vi "ATCpilot.vi"() -> ()   [LabVIEW 2014]
doc: "ATC app"
uses:
  <vilib>/Utility/config.llb/NI_LVConfig.lvlib
  <vilib>/Utility/config.llb/Read Key (String).vi
panel:
  in  "정지":bool
  in  "정보1":bool
  in  "도움말":bool
  in  "?":bool
  in  "?":bool
  in  "탭":T1(tab)
  in  "메모":string="필요한 메모를 할수 있습니다. "
  in  "SID&RadarVector. 2":string="SID&RadarVector. "
  in  "인사말":string="인사말"
  in  "CD관제기관":string="관제기관"
  in  "콜사인":string="콜사인\n콜사인\n콜사인"
  in  "도착공항":string="도착공항"
  in  "SID&RadarVector":string="SID&RadarVector"
  in  "비행고도":string="비행고도"
  in  "인사말2":string="인사말"
  in  "콜사인2":string="콜사인"
  in  "콜사인3":string="콜사인"
  in  "콜사인4":string="콜사인"
  in  "콜사인5":string="콜사인"
  in  "콜사인6":string="콜사인"
  in  "도착공항2":string="도착공항"
  in  "제한고도":string="제한고도"
  in  "비행고도2":string="비행고도"
  in  "D접속주파수":string="접속주파수"
  in  "스콱번호":string="스콱번호"
  in  "도착공항3":string="도착공항"
  in  "SID&RadarVector. 3":string="SID&RadarVector. "
  in  "제한고도2":string="제한고도"
  in  "비행고도3":string="비행고도"
  in  "D접속주파수2":string="접속주파수"
  in  "스콱번호2":string="스쾃번호"
  in  "콜사인7":string="콜사인"
  in  "콜사인8":string="콜사인"
  in  "G관제기관":string="관제기관"
  in  "G접속주파수2":string="접속주파수"
  in  "G관제기관2":string="관제기관"
  in  "G접속주파수":string="접속주파수"
  in  "콜사인9":string="콜사인"
  in  "유도로 2":string="유도로"
  in  "유도로":string="유도로"
  in  "방향 2":string="방향"
  in  "방향":string="방향"
  in  "메모2":string="필요한 메모를 할수 있습니다. "
  in  "T관제기관2":string="관제기관"
  in  "콜사인24":string="콜사인"
  in  "T접속주파수2":string="접속주파수"
  in  "T접속주파수":string="접속주파수"
  in  "T관제기관":string="관제기관"
  in  "콜사인23":string="콜사인"
  in  "활주로9":string="활주로"
  in  "G관제기관4":string="관제기관"
  in  "콜사인22":string="콜사인"
  in  "콜사인21":string="콜사인"
  in  "콜사인20":string="콜사인"
  in  "콜사인19":string="콜사인"
  in  "활주로8":string="활주로"
  in  "활주로7":string="활주로"
  in  "콜사인17":string="콜사인"
  in  "활주로6":string="활주로"
  in  "콜사인18":string="콜사인"
  in  "활주로5":string="활주로"
  in  "콜사인16":string="콜사인"
  in  "활주로4":string="활주로"
  in  "콜사인15":string="콜사인"
  in  "활주로3":string="활주로"
  in  "콜사인14":string="콜사인"
  in  "콜사인13":string="콜사인"
  in  "현재기압2":string="현재기압"
  in  "출발공항":string="출발공항"
  in  "활주로2":string="활주로"
  in  "현재기압":string="현재기압"
  in  "출발공항2":string="출발공항"
  in  "활주로1":string="활주로"
  in  "콜사인12":string="콜사인"
  in  "콜사인11":string="콜사인"
  in  "G관제기관3":string="관제기관"
  in  "인사3":string="인사"
  in  "콜사인34 2":string="콜사인"
  in  "D관제기관2":string="관제기관"
  in  "D관제기관":string="관제기관"
  in  "T관제기관3":string="관제기관"
  in  "메모3":string="필요한 메모를 할수 있습니다. "
  in  "인사4":string="인사"
  in  "콜사인25":string="콜사인"
  in  "활주로10":string="활주로"
  in  "콜사인26":string="콜사인"
  in  "바람방향":string="바람방향"
  in  "풍속":string="풍속"
  in  "콜사인28":string="콜사인"
  in  "활주로13":string="활주로"
  in  "콜사인29":string="콜사인"
  in  "활주로12":string="활주로"
  in  "콜사인30":string="콜사인"
  in  "활주로14":string="활주로"
  in  "콜사인31":string="콜사인"
  in  "활주로15":string="활주로"
  in  "T관제기관4":string="관제기관"
  in  "콜사인32":string="콜사인"
  in  "현재고도":string="현재고도"
  in  "허가고도":string="허가고도"
  in  "콜사인33":string="콜사인"
  in  "접속주파수":string="접속주파수"
  in  "콜사인34":string="콜사인"
  in  "접속주파수2":string="접속주파수"
  in  "순항고도or이니셜고도":string="순항고도or이니셜고도"
  in  "D관제기관5":string="관제기관"
  in  "메모 4":string="필요한 메모를 할수 있습니다. "
  in  "인사5":string="인사"
  in  "D관제기관3":string="관제기관"
  in  "콜사인35":string="콜사인"
  in  "현재고도A":string="현재고도"
  in  "콜사인36":string="콜사인"
  in  "D관제기관4":string="관제기관"
  in  "허가고도4":string="허가고도"
  in  "허가고도5":string="허가고도"
  in  "콜사인37":string="콜사인"
  in  "콜사인38":string="콜사인"
  in  "허가고도6":string="허가고도"
  in  "허가고도7":string="허가고도"
  in  "콜사인39":string="콜사인"
  in  "콜사인40":string="콜사인"
  in  "C관제기관":string="관제기관"
  in  "A접속주파수":string="접속주파수"
  in  "C관제기관2":string="관제기관"
  in  "A접속주파수2":string="접속주파수"
  in  "콜사인41":string="콜사인"
  in  "콜사인38 2":string="콜사인"
  in  "D관제기관6":string="관제기관"
  in  "허가고도6 2":string="허가고도"
  in  "허가고도6 3":string="허가고도"
  in  "콜사인39 2":string="콜사인"
  in  "메모5":string="필요한 메모를 할수 있습니다. "
  in  "인사말 2":string="인사말"
  in  "허가고도 2":string="허가고도"
  in  "지점":string="지점"
  in  "허가고도7 2":string="허가고도"
  in  "콜사인38 3":string="콜사인"
  in  "콜사인39 3":string="콜사인"
  in  "허가고도7 3":string="허가고도"
  in  "지점 2":string="지점"
  in  "메모6":string="필요한 메모를 할수 있습니다. "
  in  "A관제기관3":string="관제기관"
  in  "콜사인46":string="콜사인"
  in  "날시정보":string="날시정보"
  in  "고도":string="고도"
  in  "콜사인47":string="콜사인"
  in  "A관제기관4":string="관제기관"
  in  "L활주로":string="활주로"
  in  "도착공항4":string="도착공항"
  in  "현재기압":string="현재기압"
  in  "콜사인48":string="콜사인"
  in  "A관제기관5":string="관제기관"
  in  "L활주로":string="활주로"
  in  "도착공항5":string="도착공항"
  in  "현재기압":string="현재기압"
  in  "콜사인49":string="콜사인"
  in  "고도":string="고도"
  in  "콜사인50":string="콜사인"
  in  "고도":string="고도"
  in  "콜사인51":string="콜사인"
  in  "고도":string="고도"
  in  "고도":string="고도"
  in  "콜사인52":string="콜사인"
  in  "콜사인53":string="콜사인"
  in  "A관제기관":string="관제기관"
  in  "풍속":string="풍속"
  in  "바람방향":string="바람방향"
  in  "L활주로3":string="활주로"
  in  "콜사인54":string="콜사인"
  in  "L활주로":string="활주로"
  in  "콜사인55":string="콜사인"
  in  "A관제기관2":string="관제기관"
  in  "L활주로":string="활주로"
  in  "ILS":string="주파수(ils)"
  in  "콜사인56":string="콜사인"
  in  "L활주로6":string="활주로"
  in  "ILS2":string="주파수(ils)"
  in  "콜사인57":string="콜사인"
  in  "T관제기관":string="관제기관"
  in  "T접속주파수":string="접속주파수"
  in  "콜사인58":string="콜사인"
  in  "콜사인59":string="콜사인"
  in  "관제기관":string="관제기관"
  in  "T접속주파수":string="접속주파수"
  in  "메모7":string="필요한 메모를 할수 있습니다. "
  in  "바람방향":string="바람방향"
  in  "관제기관":string="관제기관"
  in  "콜사인60":string="콜사인"
  in  "L활주로7":string="활주로"
  in  "콜사인61":string="콜사인"
  in  "풍속":string="풍속"
  in  "콜사인62":string="콜사인"
  in  "L활주로":string="활주로"
  in  "L활주로":string="활주로"
  in  "관제기관":string="관제기관"
  in  "콜사인63":string="콜사인"
  in  "관제기관3":string="관제기관"
  in  "콜사인64":string="콜사인"
  in  "L활주로":string="활주로"
  in  "G관제기관":string="관제기관"
  in  "G접속주파수":string="접속주파수"
  in  "콜사인65":string="콜사인"
  in  "관제기관":string="관제기관"
  in  "G접속주파수":string="접속주파수"
  in  "콜사인70":string="콜사인"
  in  "C활주로3":string="활주로"
  in  "C활주로2":string="활주로"
  in  "관제기관3 2":string="관제기관"
  in  "C활주로":string="활주로"
  in  "콜사인69":string="콜사인"
  in  "관제기관2":string="관제기관"
  in  "메모8":string="필요한 메모를 할수 있습니다. "
  in  "관제기관":string="관제기관"
  in  "콜사인66":string="콜사인"
  in  "콜사인67":string="콜사인"
  in  "게이트번호":string="게이트번호"
  in  "THEN":string="then"
  in  "콜사인68":string="콜사인"
  in  "게이트번호2":string="게이트번호"
  in  "THEN2":string="then"
  in  "콜사인10":string="콜사인"
  in  "관제기관4":string="관제기관"
  in  "콜사인71":string="콜사인"
  in  "콜사인72":string="콜사인"
  # "pilot.v3.0"
  # "~"
  # "Good"
  # "Clearance Delivery"
  # "Pilot"
  # "at FL"
  # "Request IFR Clearance to"
  # "Airport via"
  # "~"
  # "Good"
  # "Controller"
  # ",  Clearance  Delivery, standby."
  # "Pilot"
  # "Stand by,"
  # "Controller"
  # "Delivery 또는 Delivery, Are you ready to copy?"
  # "Pilot"
  # "Go Ahead 또는 Ready to copy"
  # "Airport via"
  # ", Cleared to"
  # "Controller"
  # "ft expect FL"
  # "then as filed. Climb and Maintain"
  # "Departure Frequency"
  # "Read back."
  # "Squawk"
  # "Pilot"
  # "Airport via"
  # "Cleared to"
  # ","
  # "then as filed."
  # "Climb and Maintain"
  # "ft expect FL"
  # "Departure Frequency"
  # "and  Squawk"
  # "Controller"
  # ", Read back is corrent contact"
  # "Ground"
  # "bye bye~."
  # "Pilot"
  # "Roger, contact"
  # ", bye bye~"
  # "Pilot"
  # "Good"
  # "~"
  # "ready for push back and Engine Start."
  # ","
  # ", Rwy"
  # "Push Back and Engine Start Approved, heading to"
  # "Controller"
  # ","
  # "QNH"
  # "Read Back."
  # "Pilot"
  # "Roger\nPush Back and Engine Start Approved, heading to"
  # ", Rwy"
  # "QNH"
  # "Ready for taxi to the Rwy"
  # ","
  # "Pilot"
  # "- Push back 완료 후 -"
  # ", Ready for Taxi to Rwy"
  # "Controller"
  # ", taxi to"
  # "via taxiway"
  # ", Roger"
  # "Pilot"
  # "via taxiway"
  # "Taxi to"
  # "- 활주로를 건널 상황일 때 -"
  # "Pilot"
  # "Request Cross Rwy"
  # "Controller"
  # ", cleared Cross Rwy"
  # "Pilot"
  # "cleared Cross Rwy"
  # "Controller"
  # "Squawk Mode C."
  # "Pilot"
  # ", Roger squawk mode 'C'"
  # "------------------------ 홀딩 포인트 도착 후 ----------------------------------"
  # "Pilot"
  # "hold short of Rwy"
  # ","
  # "Controller"
  # "Roger,"
  # "contact"
  # "Tower"
  # "bye bye~"
  # "Pilot"
  # "Contact"
  # "Pilot"
  # "Good"
  # "~"
  # ",  hold short Rwy"
  # ", Ready for Departure"
  # "(곧바로 이륙허가)"
  # "Controller"
  # ", wind"
  # "knot, cleared for take off."
  # "at"
  # "(활주로 정렬대기)"
  # "Controller"
  # "Line up and wait Rwy"
  # "Pilot"
  # "Line up and wait Rwy"
  # "Roger,"
  # "(홀딩 포인트에서 대기)"
  # "Controller"
  # ", Hold short rwy"
  # ","
  # "Pilot"
  # "Hold short of Rwy"
  # "Roger,"
  # "- 이 륙 후 -"
  # "Pilot"
  # "ft."
  # "Airborn Passing"
  # "ft, Climbing"
  # ","
  # "Controller"
  # ", contact"
  # "Departure,"
  # "bye bye~"
  # "Pilot"
  # ", Roger"
  # "Contact"
  # "Departure,"
  # "bye bye~"
  # "Good"
  # "~"
  # "Pilot"
  # "Passing"
  # "expect"
  # "with (SID)."
  # ","
  # ","
  # "Controller"
  # "Departure, Radar Contact, Climb via (SID) to"
  # ","
  # "."
  # "Pilot"
  # "Roger, Climb via"
  # ","
  # "-고도제한 해제시-"
  # "Controller"
  # "Departure, Radar Contact, Climb via (SID) to"
  # ", Cancel Level Restrictions."
  # "Pilot"
  # "Roger, Climb via (SID) to"
  # ", Cancel Level Restrictions,"
  # "-속도제한 해제시-"
  # "Controller"
  # "Departure, Radar Contact, Climb via (SID) to"
  # ", Cancel Speed Restrictions."
  # "Pilot"
  # "Roger, Climb via (SID) to"
  # ", Cancel Speed Restrictions,"
  # "Controller"
  # "Control,"
  # ", bye bye."
  # ", You are leaving my airspace, Contact"
  # "Pilot"
  # "Contact"
  # "G'day"
  # "Control,"
  # ","
  # "Pilot"
  # "Good"
  # "Decend and maintain FL"
  # "with (SID)."
  # "-하강 발부-"
  # "Controller"
  # "by"
  # ", Descend and Maintain"
  # "Pilot"
  # "Descend and Maintain"
  # "by"
  # "Pilot"
  # ","
  # "FL"
  # "with information"
  # ","
  # ", Expect vector to ILS Rwy"
  # "approach"
  # "Controller"
  # "QNH"
  # "Roger,"
  # "Pilot"
  # ", Expect vector to ILS Rwy"
  # "final approach"
  # "QNH"
  # "Controller"
  # ", Decend and maintain FL"
  # "Pilot"
  # "Decend and maintain FL"
  # "Roger,"
  # "Controller"
  # ", Decend and maintain"
  # "ft"
  # "Pilot"
  # "Roger"
  # "Decend and maintain"
  # "ft"
  # "Controller"
  # ","
  # "for landing"
  # "wind"
  # "knots active Rwy"
  # "at"
  # "Pilot"
  # "Roger,"
  # "Rwy"
  # "for landing"
  # "Controller"
  # ","
  # "approach use Rwy"
  # "ILS"
  # "Roger,"
  # "Pilot"
  # "Use Rwy"
  # "ILS"
  # "- 정 렬 후 -"
  # "Pilot"
  # "Approach,"
  # ", Established on Localizer."
  # "Controller"
  # "Tower,"
  # "Good day,"
  # "Roger, Contact"
  # "Pilot"
  # "Contact"
  # "Tower"
  # "Good day,"
  # "Pilot"
  # ","
  # "Inbound Approaching Rwy"
  # "Controller"
  # ", Wind"
  # "at"
  # "knots Rwy"
  # ", Cleared to land"
  # "Pilot"
  # "Rwy"
  # "Cleared to land"
  # "Pilot"
  # ","
  # "- 착 륙 후 -"
  # ","
  # "Pilot"
  # "Touch down with Rwy"
  # "Controller"
  # "Roger, change squawk mode Standby and contact"
  # "bye bye~"
  # "ground"
  # "Pilot"
  # ", Roger"
  # "bye bye~"
  # "Change squawk mode standby and contact"
  # "- 활주로를 건널 상황일 때 -"
  # "Pilot"
  # ","
  # "Request Cross Rwy"
  # "Controller"
  # ", Cross Rwy"
  # "approved."
  # "Pilot"
  # "Cross Rwy"
  # "approved"
  # ","
  # "Pilot"
  # "Ready to taxi to the Gate"
  # "Controller"
  # ", taxi to the gate"
  # "via taxi way"
  # "Roger,"
  # "Pilot"
  # "taxi to the gate"
  # "via taxi way"
  # "- 게이트 도착 후 -"
  # "Pilot"
  # "at Gate and Engine Shut down."
  # "Thank you for your ATC service."
  # "Controller"
  # ", at the gate and Engine Shut down, Thank you ~~"
  # "Pilot"
  # "Have a nice day,"
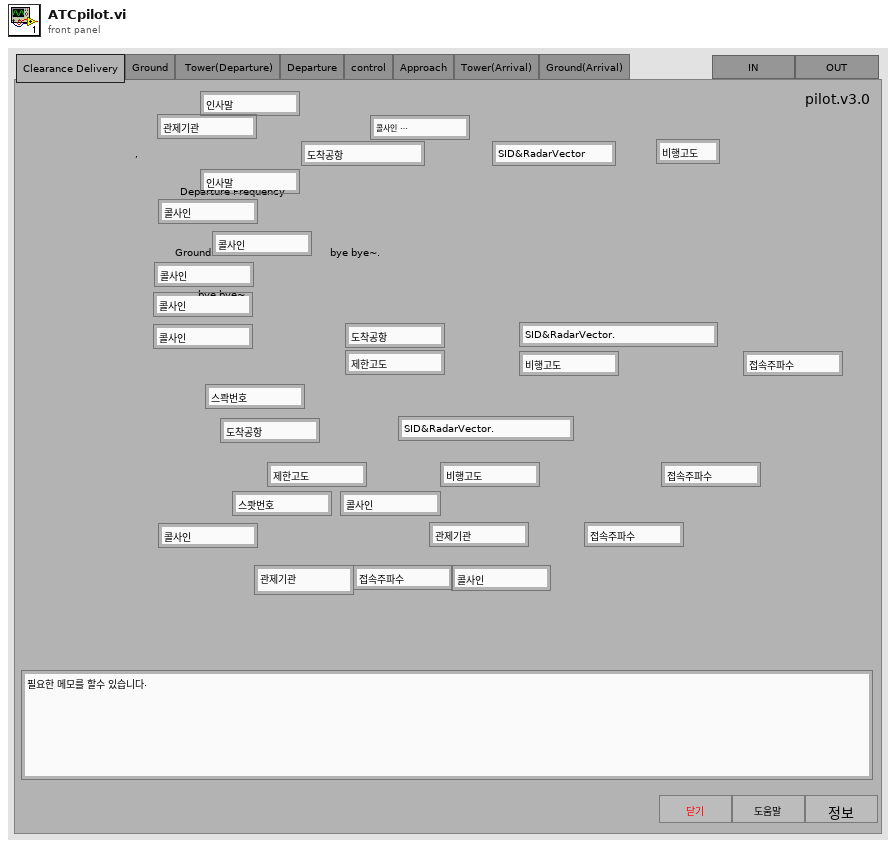
[diagram p1: front panel]
types:
  T1 = enum32{"Clearance Delivery", "Ground", " Tower(Departure)", "Departure", "control", "Approach", "Tower(Arrival)", "Ground(Arrival)"}
  T2 = typedef "NI_LVConfig.lvlib/Config Data RefNum.ctl" = refnum<k1>
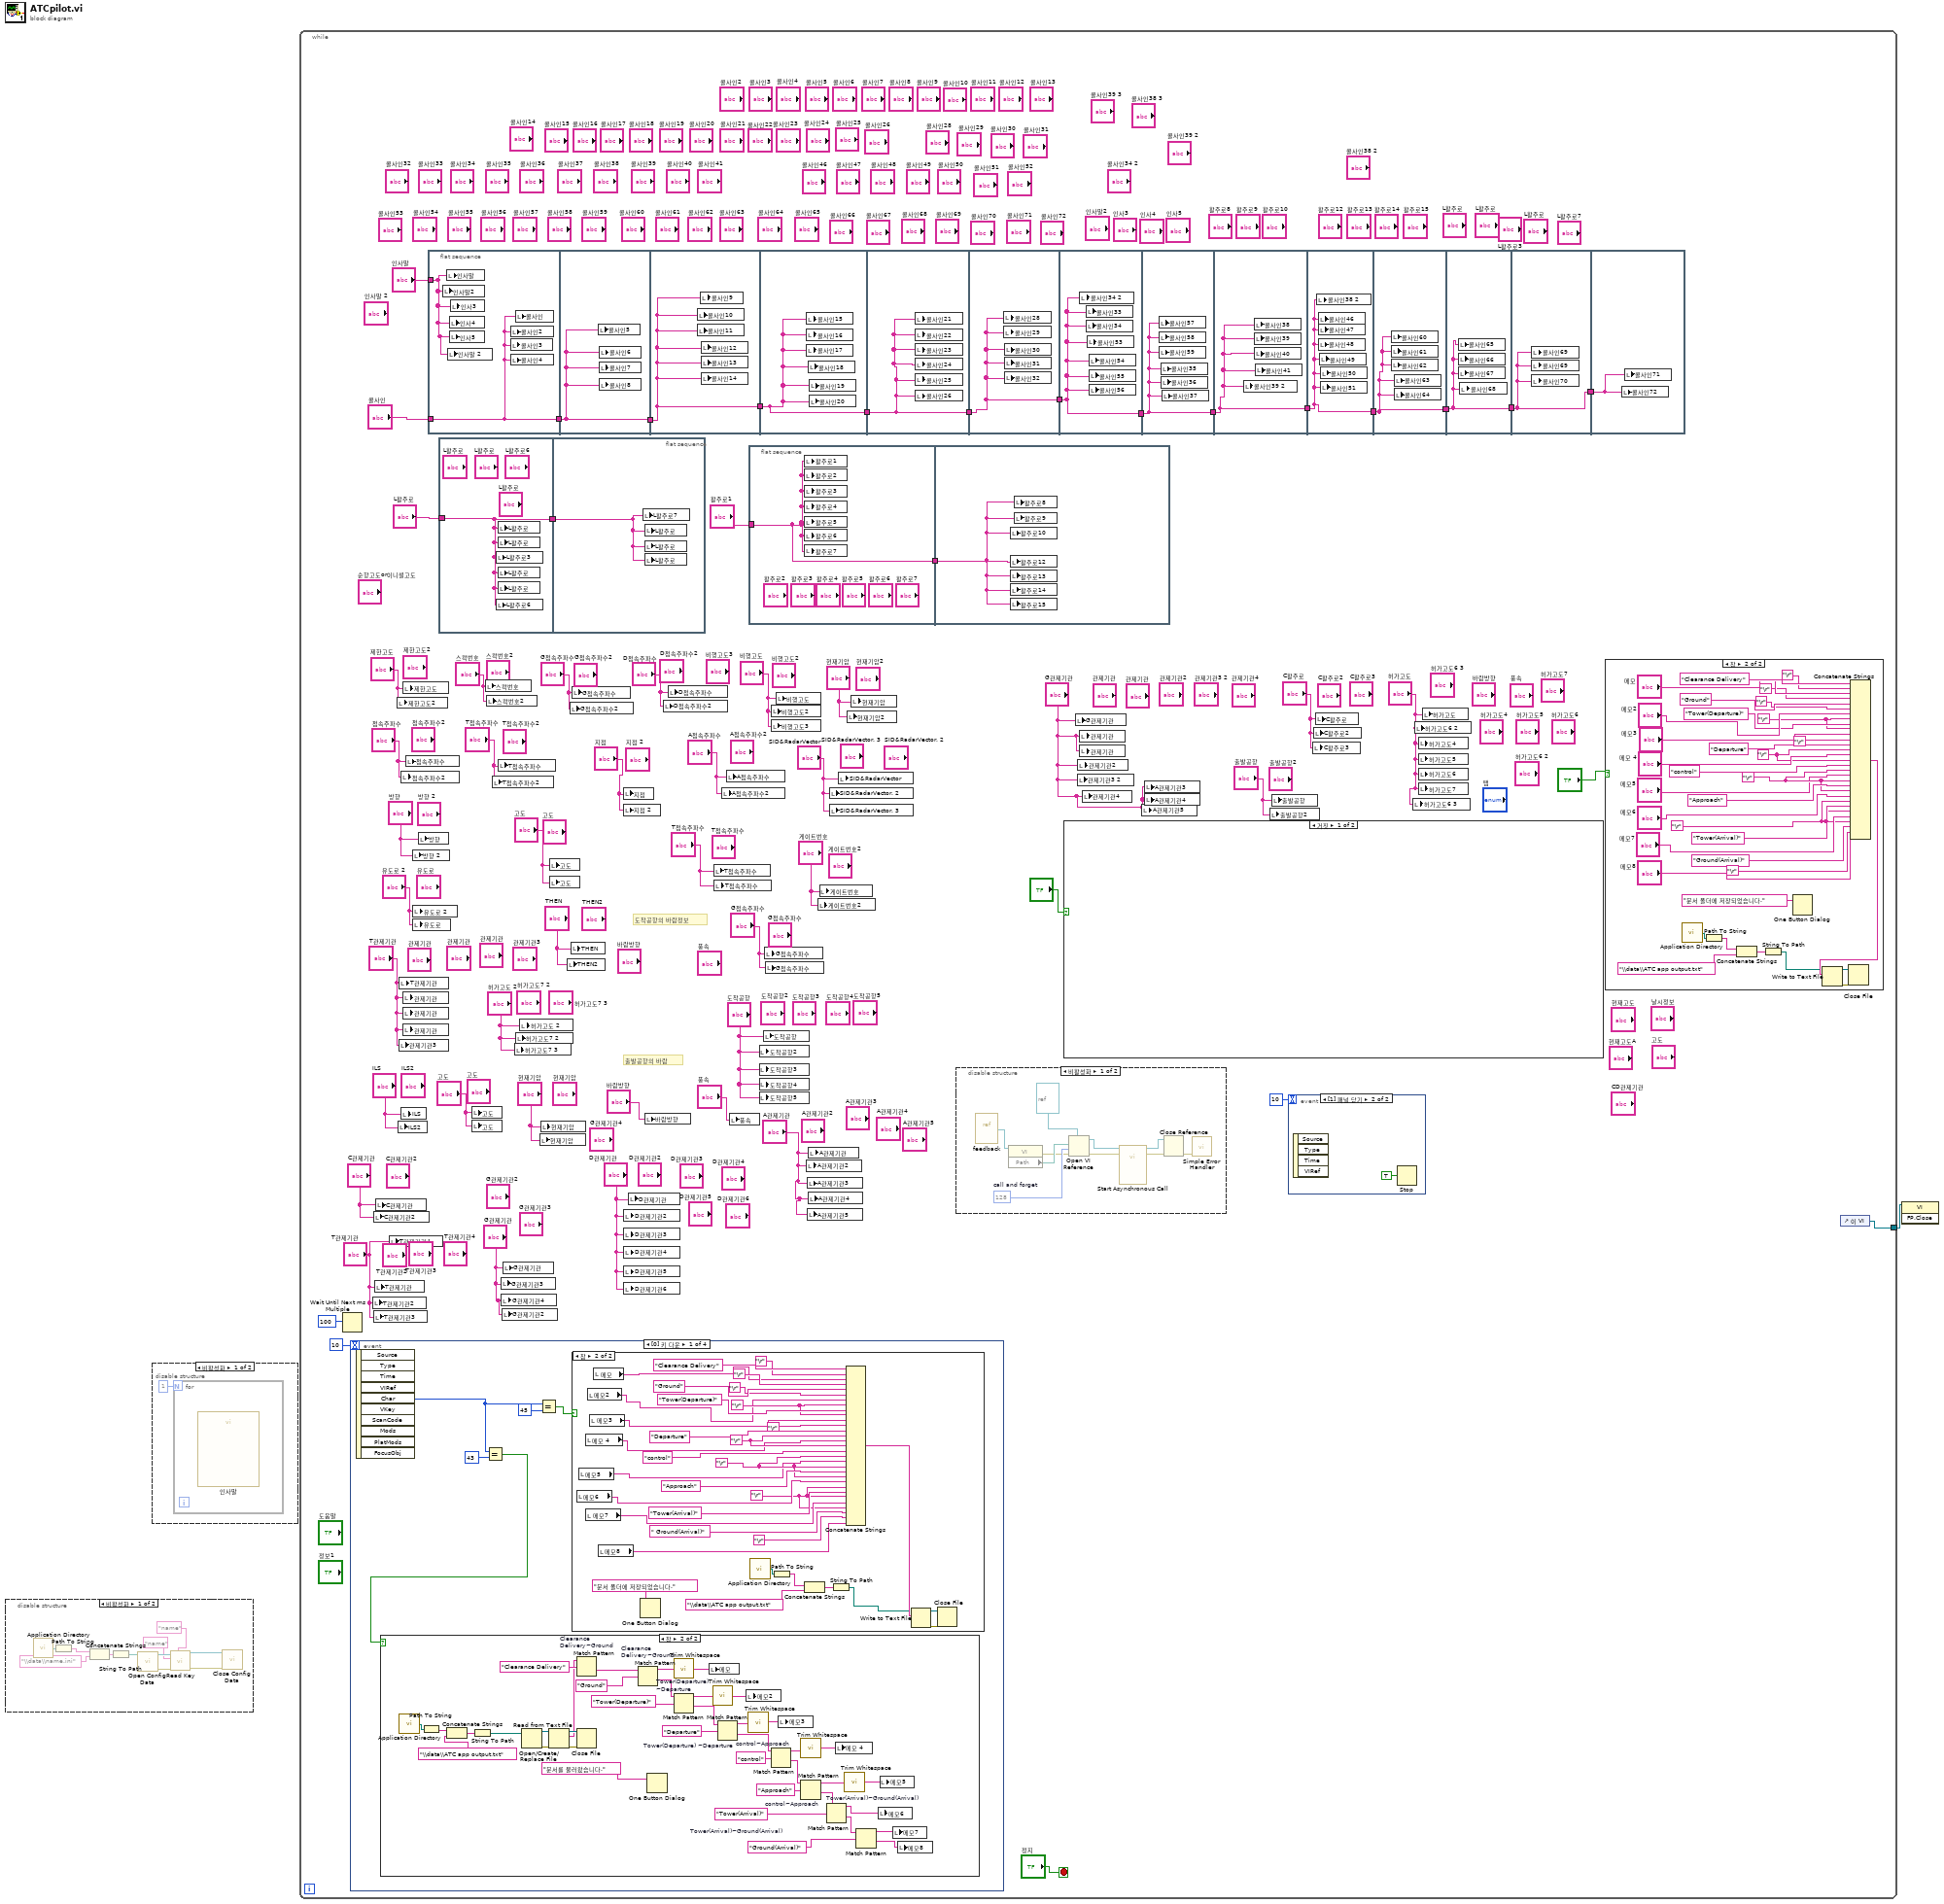
[diagram p0: block diagram]
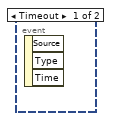
[diagram p3: hidden frame]
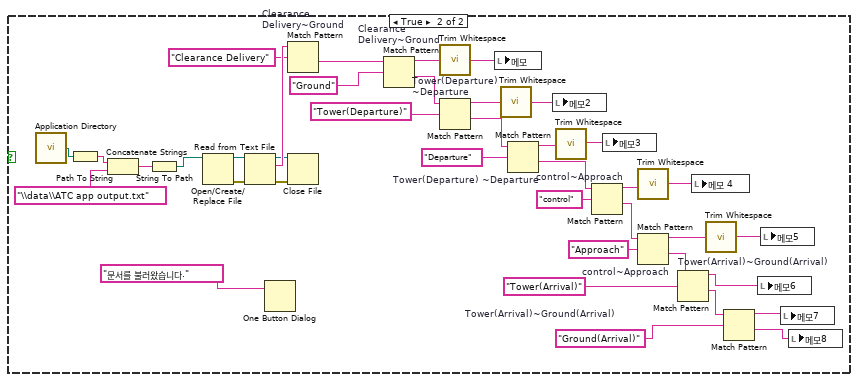
[diagram p5: hidden frame]
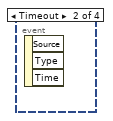
[diagram p9: hidden frame]
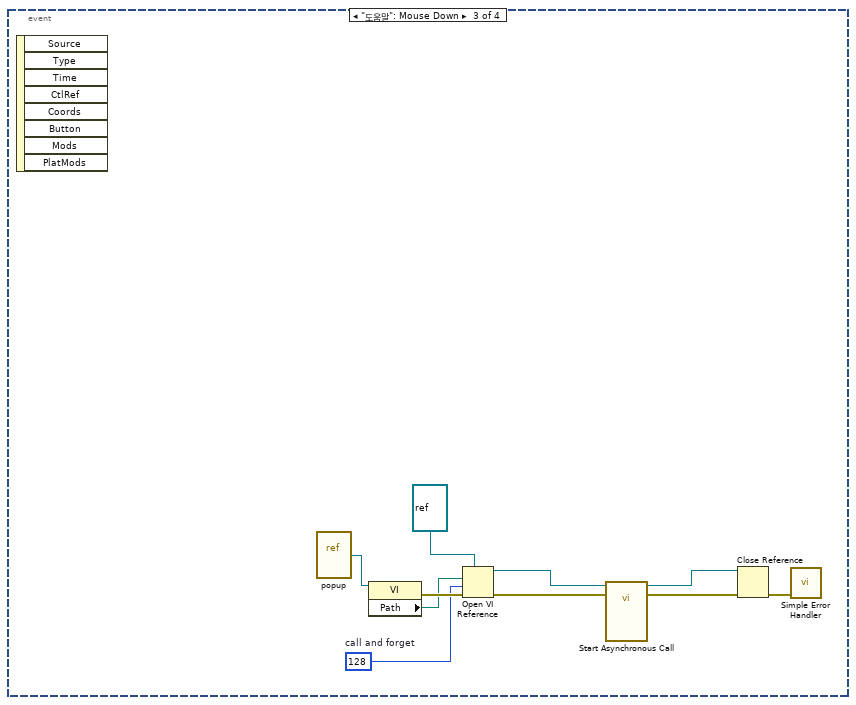
[diagram p10: hidden frame]
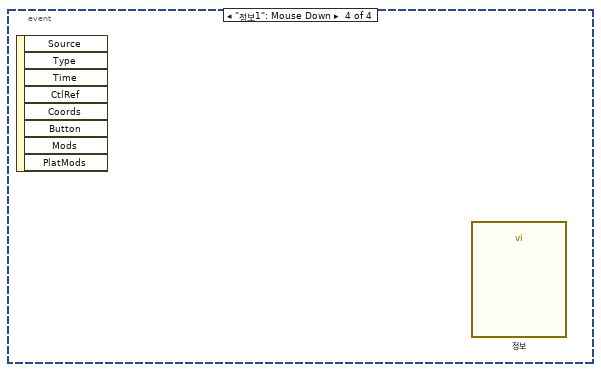
[diagram p11: hidden frame]
diagram:
  n1 = disable-structure shown="비활성화" {
    frame Disabled {
      n2 = call <vilib>:"Application Directory.vi"() -> ("Application Directory"=w2:path)
      n3 = Path To String(path=w2) -> (string=w5:string)
      n4 = Concatenate Strings(w5, "\\data\\name.ini" ("문자열")) -> (w6:string)
      n5 = String To Path(string=w6) -> (path=w4:path)
      n6 = call <vilib>:"Open Config Data.vi"("configuration file path"=w4) -> ("error out"=w11:errorcluster, "refnum"=w12:T2)  [unwired: 8 in, 1 out]
      n7 = call-poly <vilib>:"Read Key.vi"("section"="name", "error in (no error)"=w11, "key"="name", "refnum"=w12) -> ("error out"=w10:errorcluster, "refnum out"=w9:T2)  [unwired: 4 in, 2 out]
      n8 = call <vilib>:"Close Config Data.vi"("error in (no error)"=w10, "refnum"=w9) -> ()  [unwired: 8 in, 2 out]
    }
    frame Enabled {
    }
  }
  n9 = disable-structure shown="비활성화" {
    frame Disabled {
      n10 = for {
        N: 1 -> [_]
        n11 = call "인사말"() -> ()  [unwired: 10 in, 2 out]
      }
    }
    frame Enabled {
    }
  }
  n12 = while {
    tunnel: [w16] -> w1
    stop <- "정지" stop-if-true
    # "출발공항의 바람"
    # "도착공항의 바람정보"
    n13 = Wait Until Next ms Multiple(millisecond multiple=u32 100 ("대기 시간(ms)")) -> ()  [unwired: 1 out]
    n14 = event shown="[0] 키 다운" {
      selector: _ -> [_ _ _ _]
      dyn-events: _ -> [_ _ _ _]
      timeout: 10 -> [_ _ _ _]
      event Key Down {
        n15 = event-data() -> ("Char"=w179:i16)  [unwired: 1 in, 9 out]
        n16 = Equal?(x=w179, y=i16 43) -> (x = y?=w180:bool)
        n17 = case shown="참" w180 {
          frame False {
          }
          frame True {
            n18 = call <vilib>:"Application Directory.vi"() -> ("Application Directory"=w187:path)
            n19 = Path To String(path=w187) -> (string=w185:string)
            n20 = Concatenate Strings(w185, "\\data\\ATC app output.txt" ("문자열")) -> (w184:string)
            n21 = String To Path(string=w184) -> (path=w183:path)
            n22 = Open/Create/Replace File(file path (use dialog)=w183) -> (refnum out=w208:refnum<file>, error out=w207:errorcluster)  [unwired: 5 in, 1 out]
            n23 = Read from Text File(file (use dialog)=w208, error in=w207) -> (refnum out=w206:refnum<file>, text=w200:string, error out=w205:errorcluster)  [unwired: 2 in, 1 out]
            n24 = Match Pattern "Clearance Delivery~Ground"(string=w200, regular expression="Clearance Delivery" ("정규식")) -> (after substring=w203:string)  [unwired: 1 in, 3 out]
            n25 = Close File(refnum=w206, error in=w205) -> ()  [unwired: 2 out]
            n26 = Match Pattern "Clearance Delivery~Ground"(string=w203, regular expression="Ground" ("정규식")) -> (before substring=w198:string, after substring=w199:string)  [unwired: 1 in, 2 out]
            n27 = One Button Dialog(message="문서를 불러왔습니다." ("메시지")) -> ()  [unwired: 1 in, 1 out]
            n28 = call <vilib>:"Trim Whitespace.vi"("string"=w198) -> ("trimmed string"=w209:string)  [unwired: 1 in]
            n29 = Match Pattern "Tower(Departure) ~Departure"(string=w199, regular expression="Tower(Departure)" ("정규식")) -> (before substring=w197:string, after substring=w194:string)  [unwired: 1 in, 2 out]
            n30 = local write "메모"(w209) -> ()
            n31 = call <vilib>:"Trim Whitespace.vi"("string"=w197) -> ("trimmed string"=w210:string)  [unwired: 1 in]
            n32 = Match Pattern "Tower(Departure) ~Departure"(string=w194, regular expression="Departure" ("정규식")) -> (before substring=w195:string, after substring=w188:string)  [unwired: 1 in, 2 out]
            n33 = local write "메모2"(w210) -> ()
            n34 = call <vilib>:"Trim Whitespace.vi"("string"=w195) -> ("trimmed string"=w211:string)  [unwired: 1 in]
            n35 = Match Pattern "control~Approach"(string=w188, regular expression="control" ("정규식")) -> (before substring=w190:string, after substring=w192:string)  [unwired: 1 in, 2 out]
            n36 = local write "메모3"(w211) -> ()
            n37 = call <vilib>:"Trim Whitespace.vi"("string"=w190) -> ("trimmed string"=w212:string)  [unwired: 1 in]
            n38 = Match Pattern "control~Approach"(string=w192, regular expression="Approach" ("정규식")) -> (before substring=w189:string, after substring=w215:string)  [unwired: 1 in, 2 out]
            n39 = Match Pattern "Tower(Arrival)~Ground(Arrival)"(string=w215, regular expression="Tower(Arrival)" ("정규식")) -> (before substring=w217:string, after substring=w219:string)  [unwired: 1 in, 2 out]
            n40 = local write "메모 4"(w212) -> ()
            n41 = call <vilib>:"Trim Whitespace.vi"("string"=w189) -> ("trimmed string"=w213:string)  [unwired: 1 in]
            n42 = Match Pattern "Tower(Arrival)~Ground(Arrival)"(string=w219, regular expression="Ground(Arrival)" ("정규식")) -> (before substring=w220:string, after substring=w221:string)  [unwired: 1 in, 2 out]
            n43 = local write "메모6"(w217) -> ()
            n44 = local write "메모5"(w213) -> ()
            n45 = local write "메모7"(w220) -> ()
            n46 = local write "메모8"(w221) -> ()
          }
        }
        n47 = Equal?(x=w179, y=i16 45) -> (x = y?=w182:bool)
        n48 = case shown="참" w182 {
          frame False {
          }
          frame True {
            w230 = "\r"
            w242 = "\r"
            w244 = "\r"
            w247 = "\r"
            n49 = local read "메모6"() -> (w233:string)
            n50 = local read "메모5"() -> (w234:string)
            n51 = local read "메모 4"() -> (w235:string)
            n52 = local read "메모7"() -> (w231:string)
            n53 = local read "메모2"() -> (w237:string)
            n54 = local read "메모3"() -> (w236:string)
            n55 = local read "메모"() -> (w238:string)
            n56 = local read "메모8"() -> (w227:string)
            n57 = One Button Dialog(message="문서 폴더에 저장되었습니다." ("메시지")) -> ()  [unwired: 1 in, 1 out]
            n58 = call <vilib>:"Application Directory.vi"() -> ("Application Directory"=w226:path)
            n59 = Path To String(path=w226) -> (string=w224:string)
            n60 = Concatenate Strings(w224, "\\data\\ATC app output.txt" ("문자열")) -> (w223:string)
            n61 = String To Path(string=w223) -> (path=w222:path)
            n62 = Concatenate Strings("Clearance Delivery", "\r", w238, "\r", "Ground", "\r", w237, w247, "Tower(Departure)", w247, w236, "\r", "Departure", w244, w235, w244, "control", w242, w234, w242, "Approach", w242, w233, w230, "Tower(Arrival)", w230, w231, w230, " Ground(Arrival)", "\r", w227) -> (w241:string)
            n63 = Write to Text File(file (use dialog)=w222, text=w241) -> (refnum out=w255:refnum<file>, error out=w254:errorcluster)  [unwired: 2 in, 1 out]
            n64 = Close File(refnum=w255, error in=w254) -> ()  [unwired: 2 out]
          }
        }
      }
      event Timeout {
        n65 = event-data() -> ()  [unwired: 1 in, 3 out]
      }
      event "도움말": Mouse Down {
        w256 = 128  # call and forget
        n66 = event-data() -> ()  [unwired: 1 in, 8 out]
        n67 = vi-ref "popup.vi"() -> (w263:refnum<vi>)
        n68 = property class="VI"(reference=w263) -> (error out=w262:errorcluster, "Path"=w261:path)  [unwired: 1 in, 1 out]
        n69 = Open VI Reference(type specifier VI Refnum (for type only)=refnum<vi> refnum, vi path=w261, options=w256, error in (no error)=w262) -> (vi reference=w264:refnum<vi>, error out=w258:errorcluster)  [unwired: 2 in]
        n70 = call-by-ref "Start Asynchronous Call"(reference=w264, error in=w258) -> (reference out=w265:refnum<vi>, error out=w259:errorcluster)  [unwired: 12 in]
        n71 = Close Reference(reference=w265, error in (no error)=w259) -> (error out=w260:errorcluster)
        n72 = call <vilib>:"Simple Error Handler.vi"("error in (no error)"=w260) -> ()  [unwired: 4 in, 5 out]
      }
      event "정보1": Mouse Down {
        n73 = event-data() -> ()  [unwired: 1 in, 8 out]
        n74 = call "정보"() -> ()  [unwired: 10 in, 2 out]
      }
    }
    n75 = local write "T관제기관2"("T관제기관") -> ()
    n76 = local write "C관제기관2"("C관제기관") -> ()
    n77 = local write "T관제기관3"("T관제기관") -> ()
    n78 = local write "T관제기관"("T관제기관") -> ()
    n79 = local write "C관제기관"("C관제기관") -> ()
    n80 = local write "T관제기관4"("T관제기관") -> ()
    n81 = local write "제한고도2"("제한고도") -> ()
    n82 = local write "ILS2"("ILS") -> ()
    n83 = local write "관제기관3"("T관제기관") -> ()
    n84 = local write "T관제기관"("T관제기관") -> ()
    n85 = local write "접속주파수2"("접속주파수") -> ()
    n86 = local write "ILS"("ILS") -> ()
    n87 = local write "제한고도"("제한고도") -> ()
    n88 = local write "관제기관"("T관제기관") -> ()
    n89 = local write "관제기관"("T관제기관") -> ()
    n90 = local write "관제기관"("T관제기관") -> ()
    n91 = local write "접속주파수"("접속주파수") -> ()
    n92 = local write "방향 2"("방향") -> ()
    n93 = local write "유도로 2"("유도로 2") -> ()
    n94 = local write "유도로"("유도로 2") -> ()
    n95 = local write "방향"("방향") -> ()
    n96 = flat-sequence {
      tunnel: [w87] -> w64
      tunnel: "콜사인" -> [w87]
      tunnel: "인사말" -> [w86]
      tunnel: w64 -> [w88]
      tunnel: [w88] -> w63
      tunnel: w63 -> [w89]
      tunnel: [w89] -> w62
      tunnel: w62 -> [w90]
      tunnel: [w90] -> w61
      tunnel: [w91] -> w60
      tunnel: w61 -> [w91]
      tunnel: w60 -> [w92]
      tunnel: [w92] -> w59
      tunnel: [w93] -> w58
      tunnel: w59 -> [w93]
      tunnel: w58 -> [w94]
      tunnel: [w94] -> w57
      tunnel: w57 -> [w95]
      tunnel: [w95] -> w56
      tunnel: w56 -> [w96]
      tunnel: [w96] -> w55
      tunnel: w55 -> [w97]
      tunnel: [w97] -> w54
      tunnel: w54 -> [w98]
      tunnel: [w98] -> w53
      tunnel: w53 -> [w99]
      tunnel: [w99] -> w52
      tunnel: w52 -> [w100]
      frame #0 {
        n97 = local write "인사말2"(w86) -> ()
        n98 = local write "인사말"(w86) -> ()
        n99 = local write "인사말 2"(w86) -> ()
        n100 = local write "인사4"(w86) -> ()
        n101 = local write "인사5"(w86) -> ()
        n102 = local write "인사3"(w86) -> ()
        n103 = local write "콜사인3"(w87) -> ()
        n104 = local write "콜사인2"(w87) -> ()
        n105 = local write "콜사인4"(w87) -> ()
        n106 = local write "콜사인"(w87) -> ()
      }
      frame #1 {
        n107 = local write "콜사인5"(w88) -> ()
        n108 = local write "콜사인6"(w88) -> ()
        n109 = local write "콜사인7"(w88) -> ()
        n110 = local write "콜사인8"(w88) -> ()
      }
      frame #2 {
        n111 = local write "콜사인10"(w89) -> ()
        n112 = local write "콜사인11"(w89) -> ()
        n113 = local write "콜사인9"(w89) -> ()
        n114 = local write "콜사인12"(w89) -> ()
        n115 = local write "콜사인13"(w89) -> ()
        n116 = local write "콜사인14"(w89) -> ()
      }
      frame #3 {
        n117 = local write "콜사인15"(w90) -> ()
        n118 = local write "콜사인16"(w90) -> ()
        n119 = local write "콜사인17"(w90) -> ()
        n120 = local write "콜사인18"(w90) -> ()
        n121 = local write "콜사인19"(w90) -> ()
        n122 = local write "콜사인20"(w90) -> ()
      }
      frame #4 {
        n123 = local write "콜사인21"(w91) -> ()
        n124 = local write "콜사인22"(w91) -> ()
        n125 = local write "콜사인23"(w91) -> ()
        n126 = local write "콜사인24"(w91) -> ()
        n127 = local write "콜사인25"(w91) -> ()
        n128 = local write "콜사인26"(w91) -> ()
      }
      frame #5 {
        n129 = local write "콜사인28"(w92) -> ()
        n130 = local write "콜사인29"(w92) -> ()
        n131 = local write "콜사인30"(w92) -> ()
        n132 = local write "콜사인31"(w92) -> ()
        n133 = local write "콜사인32"(w92) -> ()
      }
      frame #6 {
        n134 = local write "콜사인34 2"(w93) -> ()
        n135 = local write "콜사인33"(w93) -> ()
        n136 = local write "콜사인34"(w93) -> ()
        n137 = local write "콜사인53"(w93) -> ()
        n138 = local write "콜사인54"(w93) -> ()
        n139 = local write "콜사인55"(w93) -> ()
        n140 = local write "콜사인56"(w93) -> ()
      }
      frame #7 {
        n141 = local write "콜사인57"(w94) -> ()
        n142 = local write "콜사인58"(w94) -> ()
        n143 = local write "콜사인59"(w94) -> ()
        n144 = local write "콜사인35"(w94) -> ()
        n145 = local write "콜사인36"(w94) -> ()
        n146 = local write "콜사인37"(w94) -> ()
      }
      frame #8 {
        n147 = local write "콜사인39 2"(w95) -> ()
        n148 = local write "콜사인38"(w95) -> ()
        n149 = local write "콜사인39"(w95) -> ()
        n150 = local write "콜사인40"(w95) -> ()
        n151 = local write "콜사인41"(w95) -> ()
      }
      frame #9 {
        n152 = local write "콜사인38 2"(w96) -> ()
        n153 = local write "콜사인46"(w96) -> ()
        n154 = local write "콜사인47"(w96) -> ()
        n155 = local write "콜사인48"(w96) -> ()
        n156 = local write "콜사인49"(w96) -> ()
        n157 = local write "콜사인50"(w96) -> ()
        n158 = local write "콜사인51"(w96) -> ()
      }
      frame #10 {
        n159 = local write "콜사인60"(w97) -> ()
        n160 = local write "콜사인61"(w97) -> ()
        n161 = local write "콜사인62"(w97) -> ()
        n162 = local write "콜사인63"(w97) -> ()
        n163 = local write "콜사인64"(w97) -> ()
      }
      frame #11 {
        n164 = local write "콜사인65"(w98) -> ()
        n165 = local write "콜사인66"(w98) -> ()
        n166 = local write "콜사인67"(w98) -> ()
        n167 = local write "콜사인68"(w98) -> ()
      }
      frame #12 {
        n168 = local write "콜사인69"(w99) -> ()
        n169 = local write "콜사인69"(w99) -> ()
        n170 = local write "콜사인70"(w99) -> ()
      }
      frame #13 {
        n171 = local write "콜사인72"(w100) -> ()
        n172 = local write "콜사인71"(w100) -> ()
      }
    }
    n173 = flat-sequence {
      tunnel: "L활주로" -> [w103]
      tunnel: [w103] -> w66
      tunnel: w66 -> [w104]
      frame #0 {
        n174 = local write "L활주로3"(w103) -> ()
        n175 = local write "L활주로6"(w103) -> ()
        n176 = local write "L활주로"(w103) -> ()
        n177 = local write "L활주로"(w103) -> ()
        n178 = local write "L활주로"(w103) -> ()
        n179 = local write "L활주로"(w103) -> ()
      }
      frame #1 {
        n180 = local write "L활주로7"(w104) -> ()
        n181 = local write "L활주로"(w104) -> ()
        n182 = local write "L활주로"(w104) -> ()
        n183 = local write "L활주로"(w104) -> ()
      }
    }
    n184 = local write "고도"("고도") -> ()
    n185 = local write "고도"("고도") -> ()
    n186 = local write "스콱번호"("스콱번호") -> ()
    n187 = local write "스콱번호2"("스콱번호") -> ()
    n188 = local write "T접속주파수2"("T접속주파수") -> ()
    n189 = local write "T접속주파수"("T접속주파수") -> ()
    n190 = local write "G관제기관3"("G관제기관") -> ()
    n191 = local write "G관제기관4"("G관제기관") -> ()
    n192 = local write "G관제기관2"("G관제기관") -> ()
    n193 = local write "G관제기관"("G관제기관") -> ()
    n194 = local write "허가고도7 3"("허가고도 2") -> ()
    n195 = local write "허가고도7 2"("허가고도 2") -> ()
    n196 = local write "허가고도 2"("허가고도 2") -> ()
    n197 = local write "현재기압"("현재기압") -> ()
    n198 = local write "현재기압"("현재기압") -> ()
    n199 = local write "고도"("고도") -> ()
    n200 = local write "고도"("고도") -> ()
    n201 = local write "THEN2"("THEN") -> ()
    n202 = local write "G접속주파수2"("G접속주파수") -> ()
    n203 = local write "THEN"("THEN") -> ()
    n204 = local write "G접속주파수"("G접속주파수") -> ()
    n205 = local write "지점"("지점") -> ()
    n206 = local write "지점 2"("지점") -> ()
    n207 = local write "D관제기관2"("D관제기관") -> ()
    n208 = local write "D관제기관3"("D관제기관") -> ()
    n209 = local write "D관제기관4"("D관제기관") -> ()
    n210 = local write "D관제기관5"("D관제기관") -> ()
    n211 = local write "D관제기관6"("D관제기관") -> ()
    n212 = local write "D관제기관"("D관제기관") -> ()
    n213 = local write "바람방향"("바람방향") -> ()
    n214 = local write "D접속주파수2"("D접속주파수") -> ()
    n215 = local write "D접속주파수"("D접속주파수") -> ()
    n216 = local write "T접속주파수"("T접속주파수") -> ()
    n217 = local write "T접속주파수"("T접속주파수") -> ()
    n218 = local write "A접속주파수2"("A접속주파수") -> ()
    n219 = local write "A접속주파수"("A접속주파수") -> ()
    n220 = local write "풍속"("풍속") -> ()
    n221 = flat-sequence {
      tunnel: [w101] -> w65
      tunnel: "활주로1" -> [w101]
      tunnel: w65 -> [w102]
      frame #0 {
        n222 = local write "활주로1"(w101) -> ()
        n223 = local write "활주로2"(w101) -> ()
        n224 = local write "활주로3"(w101) -> ()
        n225 = local write "활주로4"(w101) -> ()
        n226 = local write "활주로5"(w101) -> ()
        n227 = local write "활주로6"(w101) -> ()
        n228 = local write "활주로7"(w101) -> ()
      }
      frame #1 {
        n229 = local write "활주로10"(w102) -> ()
        n230 = local write "활주로12"(w102) -> ()
        n231 = local write "활주로13"(w102) -> ()
        n232 = local write "활주로14"(w102) -> ()
        n233 = local write "활주로15"(w102) -> ()
        n234 = local write "활주로8"(w102) -> ()
        n235 = local write "활주로9"(w102) -> ()
      }
    }
    n236 = local write "도착공항2"("도착공항") -> ()
    n237 = local write "도착공항3"("도착공항") -> ()
    n238 = local write "도착공항4"("도착공항") -> ()
    n239 = local write "도착공항5"("도착공항") -> ()
    n240 = local write "도착공항"("도착공항") -> ()
    n241 = local write "G접속주파수"("G접속주파수") -> ()
    n242 = local write "G접속주파수"("G접속주파수") -> ()
    n243 = local write "비행고도2"("비행고도") -> ()
    n244 = local write "비행고도3"("비행고도") -> ()
    n245 = local write "비행고도"("비행고도") -> ()
    n246 = local write "A관제기관2"("A관제기관") -> ()
    n247 = local write "A관제기관3"("A관제기관") -> ()
    n248 = local write "A관제기관5"("A관제기관") -> ()
    n249 = local write "A관제기관4"("A관제기관") -> ()
    n250 = local write "A관제기관"("A관제기관") -> ()
    n251 = local write "게이트번호2"("게이트번호") -> ()
    n252 = local write "게이트번호"("게이트번호") -> ()
    n253 = local write "SID&RadarVector. 2"("SID&RadarVector") -> ()
    n254 = local write "SID&RadarVector. 3"("SID&RadarVector") -> ()
    n255 = local write "SID&RadarVector"("SID&RadarVector") -> ()
    n256 = local write "현재기압2"("현재기압") -> ()
    n257 = local write "현재기압"("현재기압") -> ()
    n258 = disable-structure shown="비활성화" {
      frame Disabled {
        w85 = 128  # call and forget
        n259 = vi-ref "feedback.vi"() -> (w78:refnum<vi>)
        n260 = property class="VI"(reference=w78) -> (error out=w79:errorcluster, "Path"=w80:path)  [unwired: 1 in, 1 out]
        n261 = Open VI Reference(type specifier VI Refnum (for type only)=refnum<vi> refnum, vi path=w80, options=w85, error in (no error)=w79) -> (vi reference=w77:refnum<vi>, error out=w83:errorcluster)  [unwired: 2 in]
        n262 = call-by-ref "Start Asynchronous Call"(reference=w77, error in=w83) -> (reference out=w76:refnum<vi>, error out=w82:errorcluster)  [unwired: 12 in]
        n263 = Close Reference(reference=w76, error in (no error)=w82) -> (error out=w81:errorcluster)
        n264 = call <vilib>:"Simple Error Handler.vi"("error in (no error)"=w81) -> ()  [unwired: 4 in, 5 out]
      }
      frame Enabled {
      }
    }
    n265 = case shown="거짓" "?" {
      frame False {
      }
      frame True {
        n266 = call <vilib>:"Application Directory.vi"() -> ("Application Directory"=w109:path)
        n267 = Path To String(path=w109) -> (string=w107:string)
        n268 = Concatenate Strings(w107, "\\data\\ATC app output.txt" ("문자열")) -> (w106:string)
        n269 = String To Path(string=w106) -> (path=w105:path)
        n270 = Open/Create/Replace File(file path (use dialog)=w105) -> (refnum out=w123:refnum<file>, error out=w124:errorcluster)  [unwired: 5 in, 1 out]
        n271 = Read from Text File(file (use dialog)=w123, error in=w124) -> (refnum out=w125:refnum<file>, text=w131:string, error out=w126:errorcluster)  [unwired: 2 in, 1 out]
        n272 = One Button Dialog(message="문서를 불러왔습니다." ("메시지")) -> ()  [unwired: 1 in, 1 out]
        n273 = Match Pattern "Clearance Delivery~Ground"(string=w131, regular expression="Clearance Delivery" ("정규식")) -> (after substring=w128:string)  [unwired: 1 in, 3 out]
        n274 = Close File(refnum=w125, error in=w126) -> ()  [unwired: 2 out]
        n275 = Match Pattern "Clearance Delivery~Ground"(string=w128, regular expression="Ground" ("정규식")) -> (before substring=w133:string, after substring=w132:string)  [unwired: 1 in, 2 out]
        n276 = call <vilib>:"Trim Whitespace.vi"("string"=w133) -> ("trimmed string"=w122:string)  [unwired: 1 in]
        n277 = Match Pattern "Tower(Departure) ~Departure"(string=w132, regular expression="Tower(Departure)" ("정규식")) -> (before substring=w134:string, after substring=w137:string)  [unwired: 1 in, 2 out]
        n278 = local write "메모"(w122) -> ()
        n279 = call <vilib>:"Trim Whitespace.vi"("string"=w134) -> ("trimmed string"=w121:string)  [unwired: 1 in]
        n280 = Match Pattern "Tower(Departure) ~Departure"(string=w137, regular expression="Departure" ("정규식")) -> (before substring=w136:string, after substring=w143:string)  [unwired: 1 in, 2 out]
        n281 = local write "메모2"(w121) -> ()
        n282 = call <vilib>:"Trim Whitespace.vi"("string"=w136) -> ("trimmed string"=w120:string)  [unwired: 1 in]
        n283 = Match Pattern "control~Approach"(string=w143, regular expression="control" ("정규식")) -> (before substring=w141:string, after substring=w139:string)  [unwired: 1 in, 2 out]
        n284 = local write "메모3"(w120) -> ()
        n285 = call <vilib>:"Trim Whitespace.vi"("string"=w141) -> ("trimmed string"=w119:string)  [unwired: 1 in]
        n286 = Match Pattern "control~Approach"(string=w139, regular expression="Approach" ("정규식")) -> (before substring=w142:string, after substring=w116:string)  [unwired: 1 in, 2 out]
        n287 = Match Pattern "Tower(Arrival)~Ground(Arrival)"(string=w116, regular expression="Tower(Arrival)" ("정규식")) -> (before substring=w114:string, after substring=w112:string)  [unwired: 1 in, 2 out]
        n288 = local write "메모 4"(w119) -> ()
        n289 = call <vilib>:"Trim Whitespace.vi"("string"=w142) -> ("trimmed string"=w118:string)  [unwired: 1 in]
        n290 = Match Pattern "Tower(Arrival)~Ground(Arrival)"(string=w112, regular expression="Ground(Arrival)" ("정규식")) -> (before substring=w111:string, after substring=w110:string)  [unwired: 1 in, 2 out]
        n291 = local write "메모6"(w114) -> ()
        n292 = local write "메모5"(w118) -> ()
        n293 = local write "메모7"(w111) -> ()
        n294 = local write "메모8"(w110) -> ()
      }
    }
    n295 = local write "G관제기관"("G관제기관") -> ()
    n296 = local write "관제기관3 2"("G관제기관") -> ()
    n297 = local write "관제기관2"("G관제기관") -> ()
    n298 = local write "관제기관"("G관제기관") -> ()
    n299 = local write "관제기관"("G관제기관") -> ()
    n300 = local write "관제기관4"("G관제기관") -> ()
    n301 = local write "A관제기관5"("G관제기관") -> ()
    n302 = local write "A관제기관3"("G관제기관") -> ()
    n303 = local write "A관제기관4"("G관제기관") -> ()
    n304 = local write "출발공항2"("출발공항") -> ()
    n305 = local write "출발공항"("출발공항") -> ()
    n306 = event shown="[1] 패널 닫기" {
      selector: _ -> [_ _]
      dyn-events: _ -> [_ _]
      timeout: 10 -> [_ _]
      event Timeout {
        n307 = event-data() -> ()  [unwired: 1 in, 3 out]
      }
      event Panel Close {
        n308 = event-data() -> ()  [unwired: 1 in, 4 out]
        n309 = Stop(stop? (T)=TRUE ("정지? (참)")) -> ()
      }
    }
    n310 = local write "C활주로3"("C활주로") -> ()
    n311 = local write "C활주로2"("C활주로") -> ()
    n312 = local write "C활주로"("C활주로") -> ()
    n313 = local write "허가고도6 3"("허가고도") -> ()
    n314 = local write "허가고도6 2"("허가고도") -> ()
    n315 = local write "허가고도4"("허가고도") -> ()
    n316 = local write "허가고도5"("허가고도") -> ()
    n317 = local write "허가고도6"("허가고도") -> ()
    n318 = local write "허가고도7"("허가고도") -> ()
    n319 = local write "허가고도"("허가고도") -> ()
    n320 = case shown="참" "?" {
      frame False {
      }
      frame True {
        w152 = "\r"
        w159 = "\r"
        w162 = "\r"
        w167 = "\r"
        n321 = call <vilib>:"Application Directory.vi"() -> ("Application Directory"=w148:path)
        n322 = Path To String(path=w148) -> (string=w146:string)
        n323 = Concatenate Strings(w146, "\\data\\ATC app output.txt" ("문자열")) -> (w145:string)
        n324 = String To Path(string=w145) -> (path=w144:path)
        n325 = One Button Dialog(message="문서 폴더에 저장되었습니다." ("메시지")) -> ()  [unwired: 1 in, 1 out]
        n326 = Concatenate Strings("Clearance Delivery", "\r", "메모", "\r", "Ground", "\r", "메모2", w167, "Tower(Departure)", w167, "메모3", "\r", "Departure", w162, "메모 4", w162, "control", w159, "메모5", w159, "Approach", w159, "메모6", w152, "Tower(Arrival)", w152, "메모7", w152, "Ground(Arrival)", "\r", "메모8") -> (w158:string)
        n327 = Write to Text File(file (use dialog)=w144, text=w158) -> (refnum out=w177:refnum<file>, error out=w176:errorcluster)  [unwired: 2 in, 1 out]
        n328 = Close File(refnum=w177, error in=w176) -> ()  [unwired: 2 out]
      }
    }
    n329 = control-ref of="이 VI"() -> (w16:refnum<vi>)
  }
  n330 = invoke class="VI" method="FP.Close"(reference=w1) -> ()  [unwired: 2 in, 3 out]
